vi "SJ_ODE_RHS_PRESS.vi"(2 "data":T1, 3 "t":dbl, 4 "x":dbl[](array[numeric])) -> (0 "error out":errorcluster, 1 "f(x,t)":dbl[](array[numeric]))   [LabVIEW 2022 SP3]
doc: "This template is the starting point for creating a function that is the right-hand-side of an ordinary differential equaltion to be passed to the ODE Solver.vi."
uses:
  <vilib>/gmath/NumericalOptimization/objective function data.ctl
  SJ_ODE_Data.ctl
  Utilities/fluid_properties/fluid_types.ctl
  LEM_Solution_Controls.ctl
  Model.ctl
  Fourier_Series.ctl
  Utilities/fluid_properties/fluid_properties.ctl
  <vilib>/gmath/NI_Gmath.lvlib
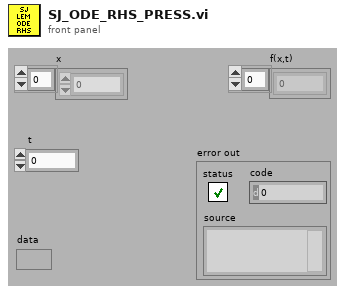
[diagram p1: front panel]
types:
  T1 = typedef "NI_Gmath.lvlib/objective function data.ctl" = variant
  T2 = typedef "SJ_ODE_Data.ctl" = cluster{"Fluid Properties":cluster{"Fluid":T3, "Temperature (K)":dbl, "Pressure (Pa)":dbl}, "SJ Geometry":cluster{"Do (mm)":dbl, "Ho (mm)":dbl, "Dc (mm)":dbl, "Hc (mm)":dbl, "Dp/Dc":dbl}, "Solution Controls":T4, "Misc Data":cluster{"Freq jet":dbl, "Coefficients":dbl[], "Nat Frequ":dbl, "Ku":dbl, "Scale":dbl, "Fourier Series":T6, "Km":dbl, "Kr":dbl}, "Thermo and Transport Properties":T7, "LEM Output Data":cluster{"X":dbl[][], "times":dbl[], "|X|":dbl, "PA X":dbl}}
  T3 = typedef "fluid_types.ctl" = enum16{"Air", "Water"}
  T4 = typedef "LEM_Solution_Controls.ctl" = cluster{"Simulation":enum16{"Sinusoidal", "Fourier Series"}, "Fixed Parameter":enum16{"Pressure", "Displacement"}, "Model":T5, "# time steps":i32, "# periods":i32, "Tolerance":dbl, "STFT periods":i32}
  T5 = typedef "Model.ctl" = enum16{"Martin", "Tang", "Gallas", "Persoon"}
  T6 = typedef "Fourier_Series.ctl" = cluster{"Amp":dbl, "Phase":dbl}[]
  T7 = typedef "fluid_properties.ctl" = cluster{"nu":dbl, "c":dbl, "Pr":dbl, "Cp":dbl, "Cv":dbl, "gamma":dbl, "mu":dbl, "rho":dbl}
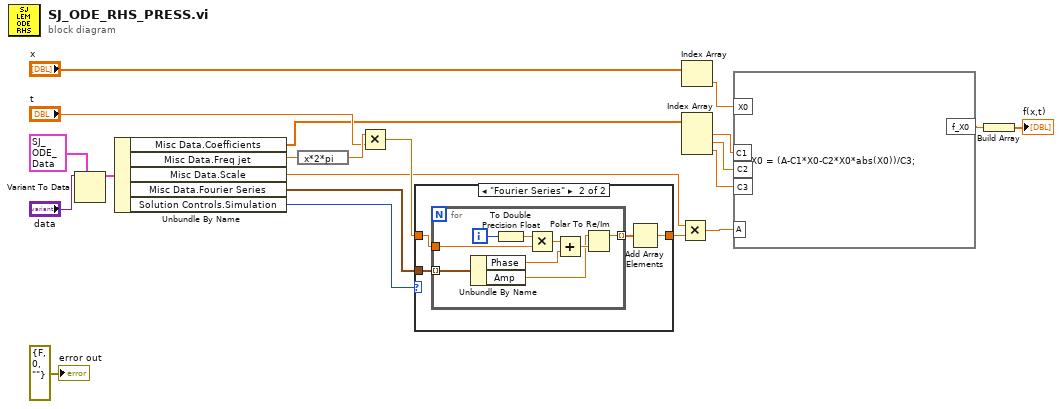
[diagram p0: block diagram]
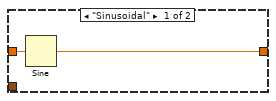
[diagram p2: hidden frame]
diagram:
  n1 = Variant To Data(type=T2 {"Fluid Properties"={"Fluid"=enum."Air", "Temperature (K)"=0.0, "Pressure (Pa)"=0.0}, "SJ Geometry"={"Do (mm)"=0.0, "Ho (mm)"=0.0, "Dc (mm)"=0.0, "Hc (mm)"=0.0, "Dp/Dc"=6.5}, "Solution Controls"={"Simulation"=enum."Sinusoidal", "Fixed Parameter"=enum."Pressure", "Model"=enum."Tang", "# time steps"=0, "# periods"=0, "Tolerance"=0.0, "STFT periods"=0}, "Misc Data"={"Freq jet"=0.0, "Coefficients"=[], "Nat Frequ"=0.0, "Ku"=0.0, "Scale"=0.0, "Fourier Series"=[], "Km"=0.0, "Kr"=0.0}, "Thermo and Transport Properties"={"nu"=0.0, "c"=0.0, "Pr"=0.0, "Cp"=0.0, "Cv"=0.0, "gamma"=0.0, "mu"=0.0, "rho"=0.0}, "LEM Output Data"={"X"=[], "times"=[], "|X|"=0.0, "PA X"=0.0}} ("ODE Data"), Variant="data") -> (data=w9:T2)  [unwired: 1 in, 1 out]
  n2 = Unbundle By Name(w9) -> ("Misc Data.Coefficients"=w6:dbl[], "Misc Data.Freq jet"=w10:dbl, "Misc Data.Scale"=w2:dbl, "Misc Data.Fourier Series"=w3:T6, "Solution Controls.Simulation"=w4:enum16{"Sinusoidal", "Fourier Series"})
  n3 = expression code="x*2*pi"(w10) -> (w11:dbl)
  n4 = Multiply(x=w11, y="t") -> (x*y=w5:dbl)
  n5 = case shown="\"Fourier Series\"" w4 {
    tunnel: w5 -> [w23 w26]
    tunnel: [w22 w24] -> w1
    tunnel: w3 -> [_ w27]
    frame "Sinusoidal" {
      n6 = Sine(x=w23) -> (sin(x)=w22:dbl)
    }
    frame "Fourier Series" {
      n7 = for {
        tunnel: w27 -> [w34] mode=indexing
        tunnel: w26 -> [w35]
        tunnel: [w29] -> w25 mode=indexing
        i -> [w30]
        n8 = Unbundle By Name(w34) -> ("Phase"=w32:dbl, "Amp"=w28:dbl)
        n9 = To Double Precision Float(number=w30) -> (double precision float=w36:dbl)
        n10 = Multiply(x=w36, y=w35) -> (x*y=w33:dbl)
        n11 = Add(x=w33, y=w32) -> (x+y=w31:dbl)
        n12 = Polar To Re/Im(2:w31, 3:w28) -> (1:w29:dbl)  [unwired: 1 out]
      }
      n13 = Add Array Elements(numeric array=w25) -> (sum=w24:dbl)
    }
  }
  n14 = Multiply(x=w2, y=w1) -> (x*y=w7:dbl)
  n15 = Index Array(array="x") -> (element=w17:dbl)  [unwired: 1 in]
  n16 = Index Array(array=w6) -> (element #1=w14:dbl, element #2=w13:dbl, element #3=w12:dbl)  [unwired: 3 in]
  n17 = formula code="f_X0 = (A-C1*X0-C2*X0*abs(X0))/C3;"("C1"=w14, "C2"=w13, "C3"=w12, "X0"=w17, "A"=w7) -> ("f_X0"=w16:dbl)
  n18 = Build Array(w16) -> (→"f(x,t)":dbl[])
  "error out" <- errorcluster {"status"=FALSE, "code"=0, "source"=""} ("error out")
